vi "configuration setup.vi"(0 "IMAQdx Session":T1, 1 "VideoMode":u32, 2 "Gain":u32, 3 "Gamma":dbl, 4 "Contrast":dbl, 5 "Exposure":u32, 6 "Saturation":u32, 7 "error in (no error)":errorcluster) -> (20 "IMAQdx Session 2":T1, 27 "error out":errorcluster)   [LabVIEW 2016, in "CCD.lvlib" / "CCD.lvclass"]
uses:
  <userlib>/Common Components/Hardware/CCD/CCD/CCD.lvclass
  <vilib>/userdefined/High Color/IMAQdx.ctl
  <resource>/objmgr/imaqdx.rc
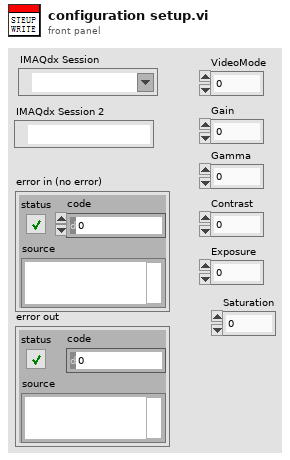
[diagram p1: front panel]
types:
  T1 = typedef "IMAQdx.ctl" = refnum<k21>
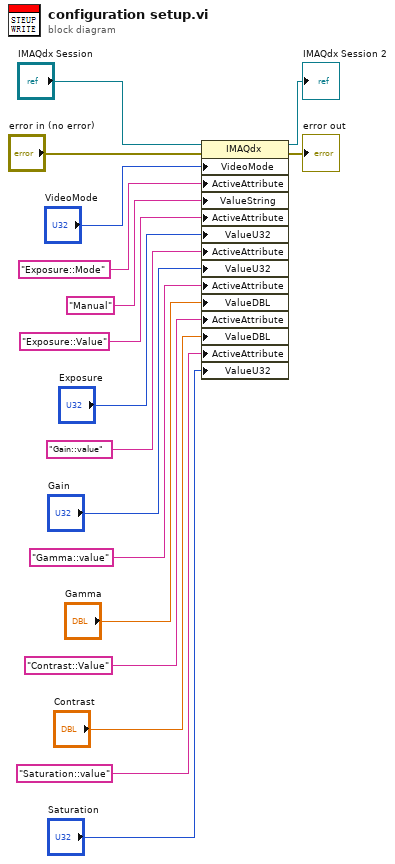
[diagram p0: block diagram]
diagram:
  n1 = property class="IMAQdx"(reference="IMAQdx Session", error in="error in (no error)", "VideoMode"="VideoMode", "ActiveAttribute"="Exposure::Mode", "ValueString"="Manual", "ActiveAttribute"="Exposure::Value", "ValueU32"="Exposure", "ActiveAttribute"="Gain::value", "ValueU32"="Gain", "ActiveAttribute"="Gamma::value", "ValueDBL"="Gamma", "ActiveAttribute"="Contrast::Value", "ValueDBL"="Contrast", "ActiveAttribute"="Saturation::value", "ValueU32"="Saturation") -> (reference out=→"IMAQdx Session 2":T1, error out=→"error out":errorcluster)
